vi "PAUSE.vi"() -> ()   [LabVIEW 2015]
uses:
  Global.vi
panel:
  in  "stop":bool
  out "VAR index":i32
  out "Val":u32=4000
  out "Old_Val":u32=4000
  out "Set":bool
  out "Recieved":bool
  in  "Var":string="PAUSE"
  # "Wait (ms).\n\nValue Type: U32\nOptions: none"
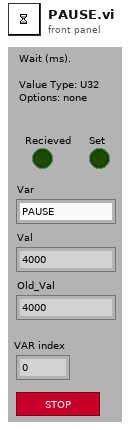
[diagram p1: front panel]
types:
  T1 = typedef "Semaphore RefNum" = refnum<k1>
  T2 = cluster{"VAR":string, "Options":string, "Val":string, "Recieved":bool, "Set":bool}[]
  T3 = cluster{"VAR":string, "Options":string, "Val":string, "Recieved":bool, "Set":bool}
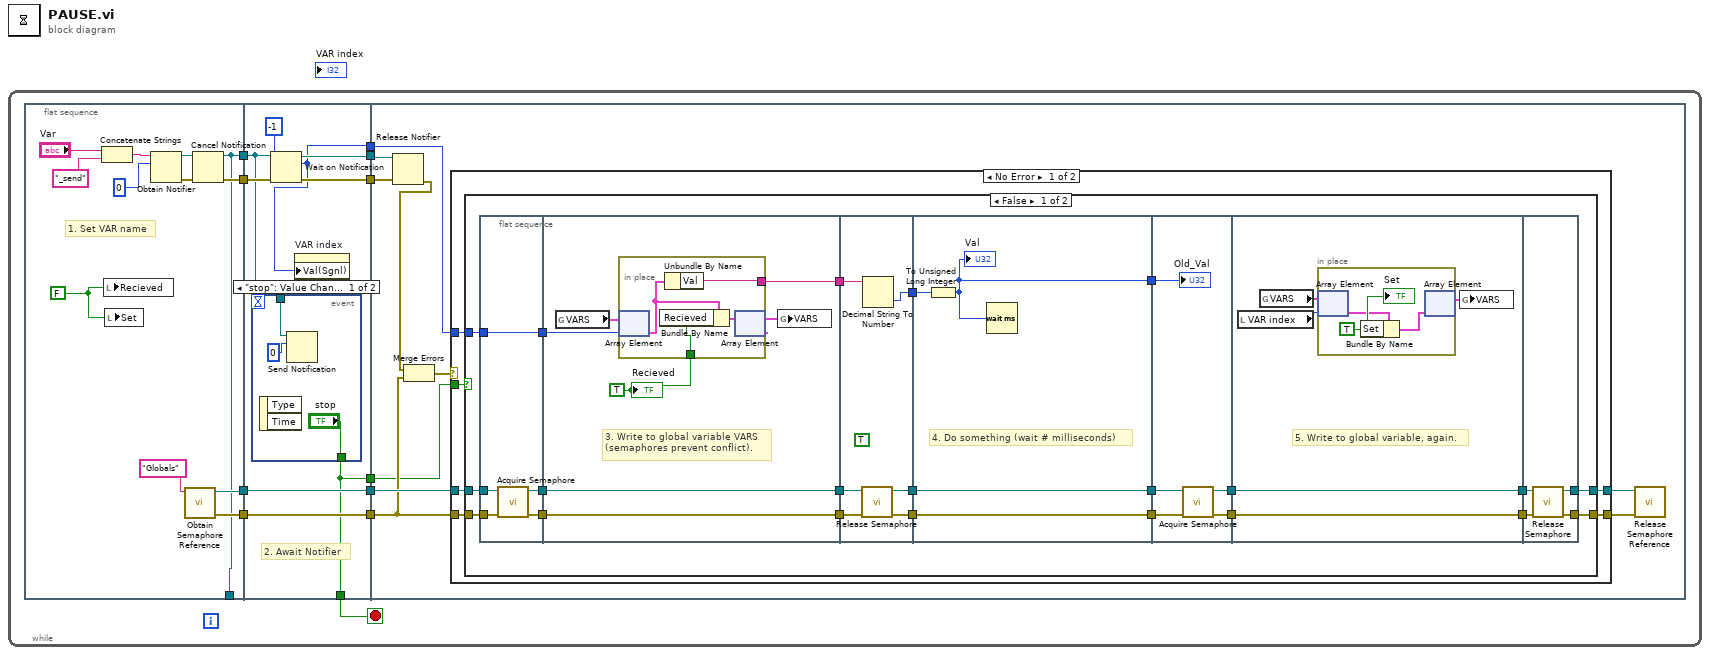
[diagram p0: block diagram]
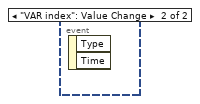
[diagram p2: hidden frame]
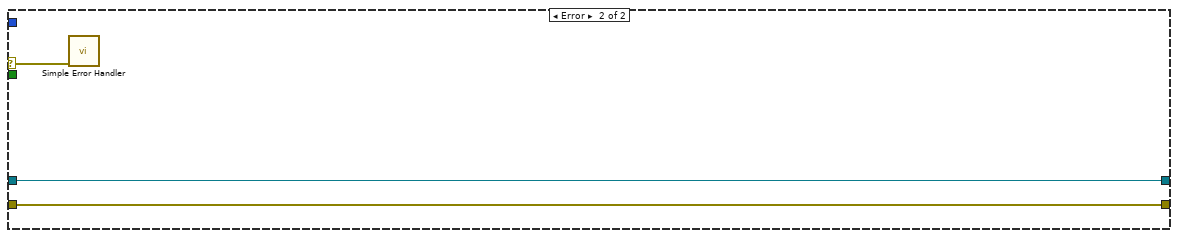
[diagram p4: hidden frame]
diagram:
  n1 = while {
    stop <- w2 stop-if-true
    n2 = flat-sequence {
      tunnel: [w14] -> w11
      tunnel: [w13] -> w10
      tunnel: [w21] -> w6
      tunnel: [w20] -> w4
      tunnel: [w13] -> _
      tunnel: w11 -> [w31]
      tunnel: w10 -> [w25]
      tunnel: [w30] -> w9
      tunnel: [w27] -> w8
      tunnel: [w26] -> w7
      tunnel: w6 -> [w29]
      tunnel: [w29] -> w5
      tunnel: w4 -> [w28]
      tunnel: [w28] -> w3
      tunnel: [w24] -> w2
      tunnel: [w24] -> w1
      tunnel: w9 -> [w38]
      tunnel: w8 -> [w39]
      tunnel: w7 -> [w45]
      tunnel: w5 -> [w44]
      tunnel: w3 -> [w41]
      tunnel: w1 -> [w36]
      frame #0 {
        w23 = FALSE ("notification")
        # "1. Set VAR name"
        n3 = Concatenate Strings("Var", "_send") -> (w18:string)
        n4 = local write "Recieved"(w23) -> ()
        n5 = local write "Set"(w23) -> ()
        n6 = Obtain Notifier(name (unnamed)=w18, notification data type=0) -> (notifier out=w12:refnum<notifier>, error out=w15:errorcluster)  [unwired: 2 in, 1 out]
        n7 = call <vilib>:"Obtain Semaphore Reference.vi"("name (unnamed)"="Globals") -> ("error out"=w20:errorcluster, "semaphore"=w21:T1)  [unwired: 4 in, 1 out]
        n8 = Cancel Notification(0:w12, 3:w15) -> (8:w13:refnum<notifier>, 11:w14:errorcluster)  [unwired: 1 out]
      }
      frame #1 {
        # "2. Await Notifier"
        n9 = event shown="[0] \"stop\": Value Change" {
          selector: _ -> [_ _]
          dyn-events: _ -> [_ _]
          timeout: _ -> [_ _]
          tunnel: ["stop" _] -> w24
          tunnel: w25 -> [w34 _]
          event "stop": Value Change {
            n10 = event-data() -> ()  [unwired: 1 in, 2 out]
            n11 = Send Notification(notification=0, notifier=w34) -> ()  [unwired: 1 in, 2 out]
          }
          event "VAR index": Value Change {
            n12 = event-data() -> ()  [unwired: 1 in, 2 out]
          }
        }
        n13 = Wait on Notification(notifier=w25, timeout in ms (-1)=-1, error in (no error)=w31) -> (notifier out=w30:refnum<notifier>, notification=w26:i32, error out=w27:errorcluster)  [unwired: 1 in, 1 out]
        n14 = property on="VAR index" class="DigNum (strict)"("Val(Sgnl)"=w26) -> ()  [unwired: 2 in, 2 out]
      }
      frame #2 {
        n15 = Release Notifier(notifier=w38, error in (no error)=w39) -> (error out=w37:errorcluster)  [unwired: 1 in, 2 out]
        n16 = Merge Errors(w37, w41) -> (w40:errorcluster)
        n17 = case shown="No Error" w40 {
          selector: w40 -> [_ w118]
          tunnel: w45 -> [w51 _]
          tunnel: w44 -> [w50 w120]
          tunnel: w41 -> [w49 w119]
          tunnel: [w48 w119] -> w43
          tunnel: [w47 w120] -> w42
          tunnel: w36 -> [w46 _]
          frame No Error {
            n18 = case shown="False" w46 {
              tunnel: w51 -> [w57 _]
              tunnel: w50 -> [w56 w117]
              tunnel: w49 -> [w55 w116]
              tunnel: [w54 w116] -> w48
              tunnel: [w53 w117] -> w47
              frame False {
                n19 = flat-sequence {
                  tunnel: w55 -> [w75]
                  tunnel: w56 -> [w76]
                  tunnel: w57 -> [w77]
                  tunnel: [w77] -> w72
                  tunnel: [w74] -> w71
                  tunnel: [w73] -> w70
                  tunnel: w72 -> [w79]
                  tunnel: w71 -> [w83]
                  tunnel: w70 -> [w84]
                  tunnel: [w84] -> w69
                  tunnel: [w83] -> w68
                  tunnel: [w78] -> w67
                  tunnel: w69 -> [w93]
                  tunnel: w68 -> [w94]
                  tunnel: [w92] -> w66
                  tunnel: [w91] -> w65
                  tunnel: [w89] -> w64
                  tunnel: w67 -> [w90]
                  tunnel: w66 -> [w98]
                  tunnel: w65 -> [w97]
                  tunnel: [w98] -> w63
                  tunnel: [w97] -> w62
                  tunnel: w64 -> [w96]
                  tunnel: [w95] -> w52
                  tunnel: w63 -> [w103]
                  tunnel: w62 -> [w100]
                  tunnel: [w102] -> w61
                  tunnel: [w101] -> w60
                  tunnel: w52 -> [w99]
                  tunnel: [w108] -> w59
                  tunnel: w61 -> [w108]
                  tunnel: [w104] -> w58
                  tunnel: w60 -> [w104]
                  tunnel: w59 -> [w115]
                  tunnel: w58 -> [w114]
                  tunnel: [w113] -> w54
                  tunnel: [w112] -> w53
                  frame #0 {
                    n20 = call <vilib>:"Acquire Semaphore.vi"("error in (no error)"=w75, "semaphore"=w76) -> ("error out"=w74:errorcluster, "semaphore out"=w73:T1)  [unwired: 3 in, 1 out]
                  }
                  frame #1 {
                    w80 = TRUE ("Found")
                    # "3. Write to global variable VARS\n(semaphores prevent conflict)."
                    n21 = global read "Global.vi" "VARS"() -> (w81:T2)
                    n22 = in-place {
                      in-place-border: [w86] -> w78
                      in-place-border: w80 -> [w85]
                      n23 = in-place-array #1(w81, w79) -> (w88:T3)
                      n24 = Bundle By Name(cluster=w88, "Recieved"=w85) -> (w87:T3)
                      n25 = Unbundle By Name(w88) -> ("Val"=w86:string)
                      n26 = in-place-array #1(w87) -> (w82:T2)  [unwired: 1 out]
                    }
                    n27 = global write "Global.vi" "VARS"(w82) -> ()
                    "Recieved" <- w80
                  }
                  frame #2 {
                    (unwired) TRUE ("Blinking")
                    n28 = call <vilib>:"Release Semaphore.vi"("error in (no error)"=w94, "semaphore"=w93) -> ("error out"=w91:errorcluster, "semaphore out"=w92:T1)  [unwired: 4 in]
                    n29 = Decimal String To Number(string=w90) -> (number=w89:i32)  [unwired: 2 in, 1 out]
                  }
                  frame #3 {
                    # "4. Do something (wait # milliseconds)"
                    n30 = To Unsigned Long Integer(number=w96) -> (unsigned 32bit integer=w95:u32)
                    "Val" <- w95
                    n31 = Wait (ms)(milliseconds to wait=w95) -> ()  [unwired: 1 out]
                  }
                  frame #4 {
                    n32 = call <vilib>:"Acquire Semaphore.vi"("error in (no error)"=w100, "semaphore"=w103) -> ("error out"=w101:errorcluster, "semaphore out"=w102:T1)  [unwired: 3 in, 1 out]
                    "Old_Val" <- w99
                  }
                  frame #5 {
                    # "5. Write to global variable, again."
                    n33 = local read "VAR index"() -> (w107:i32)
                    n34 = global read "Global.vi" "VARS"() -> (w106:T2)
                    n35 = in-place {
                      w111 = TRUE ("Set")
                      n36 = in-place-array #2(w106, w107) -> (w110:T3)
                      n37 = Bundle By Name(cluster=w110, "Set"=w111) -> (w109:T3)
                      n38 = in-place-array #2(w109) -> (w105:T2)  [unwired: 1 out]
                      "Set" <- w111
                    }
                    n39 = global write "Global.vi" "VARS"(w105) -> ()
                  }
                  frame #6 {
                    n40 = call <vilib>:"Release Semaphore.vi"("error in (no error)"=w114, "semaphore"=w115) -> ("error out"=w113:errorcluster, "semaphore out"=w112:T1)  [unwired: 4 in]
                  }
                }
              }
              frame True {
              }
            }
          }
          frame Error {
            n41 = call <vilib>:"Simple Error Handler.vi"("error in (no error)"=w118) -> ()  [unwired: 4 in, 5 out]
          }
        }
        n42 = call <vilib>:"Release Semaphore Reference.vi"("error in (no error)"=w43, "semaphore"=w42) -> ()  [unwired: 8 in, 2 out]
      }
    }
  }
